vi "Create RT FIFO.vi"(8 "error in (no error)":errorcluster) -> (0 "error out":errorcluster, 2 "RT FIFO":refnum<k33>)   [LabVIEW 2024]
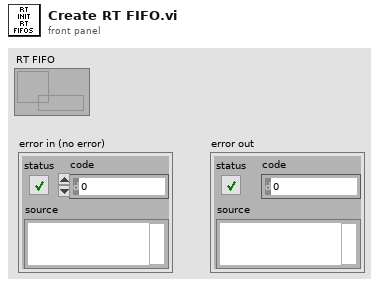
[diagram p1: front panel]
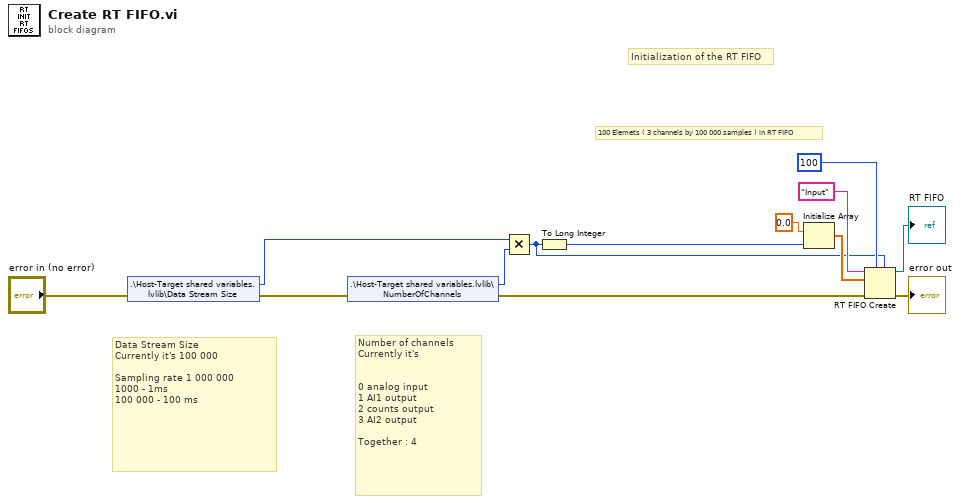
[diagram p0: block diagram]
diagram:
  # "Initialization of the RT FIFO"
  # "Data Stream Size\nCurrently it's 100 000\n\nSampling rate 1 000 000\n1000 - 1ms\n100 000 - 100 ms"
  # "100 Elemets ( 3 channels by 100 000 samples ) in RT FIFO"
  # "Number of channels\nCurrently it's\n\n\n0 analog input \n1 AI1 output\n2 counts output\n3 AI2 output\n\nTogether : 4"
  n1 = shared-variable ".\\Host-Target shared variables.lvlib\\Data Stream Size"(error in="error in (no error)") -> (w1:u32, error out=w2:errorcluster)
  n2 = shared-variable ".\\Host-Target shared variables.lvlib\\NumberOfChannels"(error in=w2) -> (w5:u8, error out=w4:errorcluster)
  n3 = Multiply(x=w1, y=w5) -> (x*y=w7:u32)
  n4 = To Long Integer(number=w7) -> (32bit integer=w6:i32)
  n5 = Initialize Array(sgl 0.0, w6) -> (w10:sgl[])
  n6 = RT FIFO Create(0:"Input" ("name (unnamed)"), 1:w10, 3:w4, 4:u32 100 ("size (10)"), 6:w7) -> (8:→"RT FIFO":refnum<k33>, 11:→"error out":errorcluster)  [unwired: 3 in, 1 out]
